vi "test Caller Stop on Last Ack.vi"(8 "error in (no error)":errorcluster, 11 "TestCase in":refnum<class "Test TCP Caller Endpoint Disconnect.lvclass">) -> (0 "error out":errorcluster, 3 "TestCase out":refnum<class "Test TCP Caller Endpoint Disconnect.lvclass">)   [LabVIEW 2020, in "Test TCP Caller Endpoint Disconnect.lvclass"]
uses:
  Test TCP Caller Endpoint Disconnect.lvclass
  <vilib>/addons/_JKI Toolkits/VI Tester/TestCase.llb/TestCase.lvclass
  <vilib>/ActorFramework/Message Queue/Message Queue.lvclass
  <vilib>/ActorFramework/LastAck/Last Ack.lvclass
  <vilib>/ActorFramework/Message Dequeuer/Message Dequeuer.lvclass
  Support/Caller Test Harness/Caller Test Harness Messages/Write String Data Msg/Write String Data Msg.lvclass
  Source/Caller Endpoint/Caller Endpoint/Caller Endpoint.lvclass
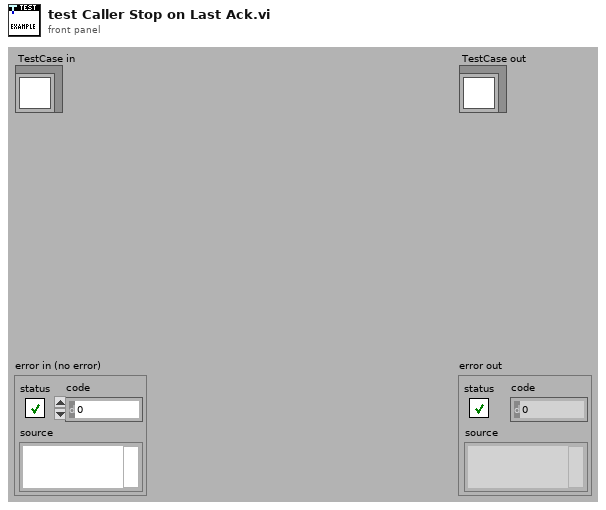
[diagram p1: front panel]
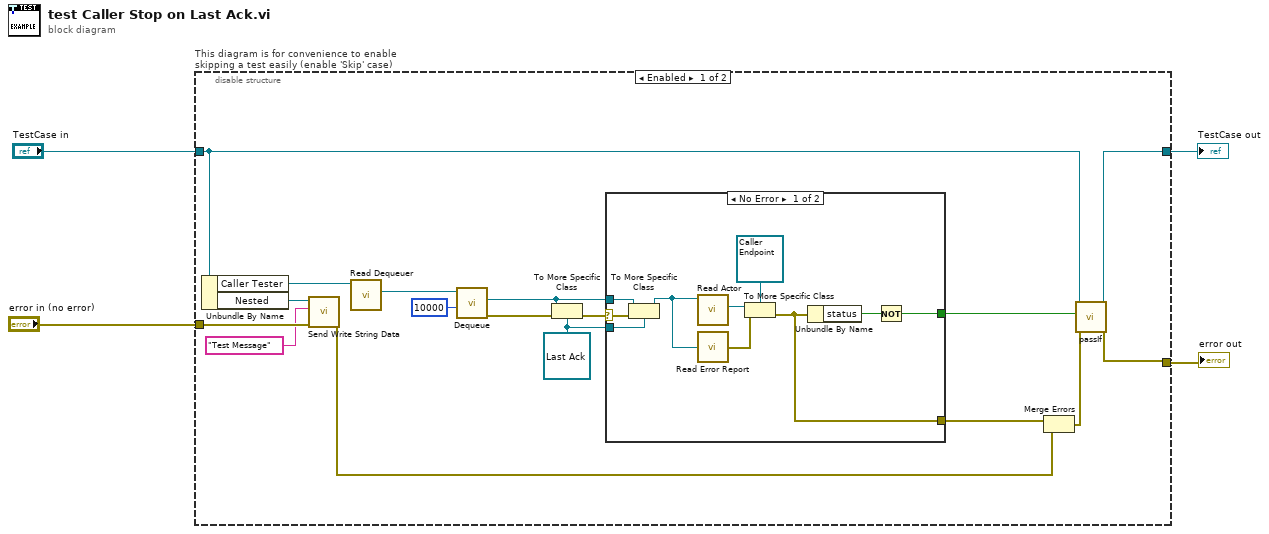
[diagram p0: block diagram]
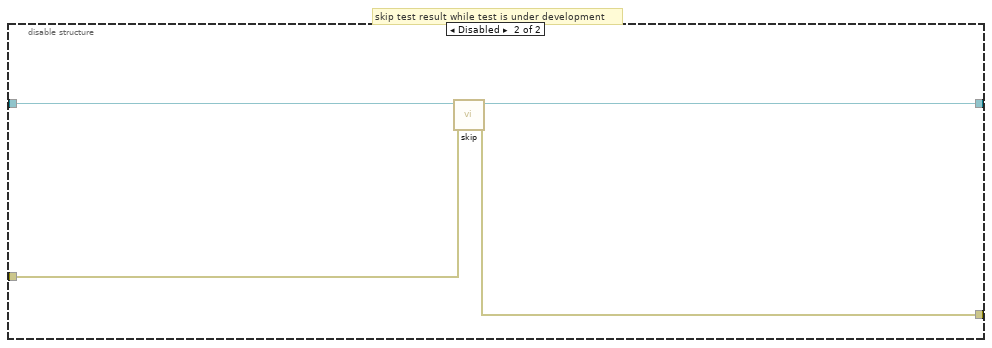
[diagram p3: hidden frame]
diagram:
  n1 = disable-structure "This diagram is for convenience to enable skipping a test easily (enable 'Skip' case)" shown="Enabled" {
    disable-tunnel: "TestCase in" -> [w19 w35]
    disable-tunnel: [w21 w33] -> w1
    disable-tunnel: [w20 w34] -> w3
    disable-tunnel: "error in (no error)" -> [w13 w32]
    frame Enabled {
      w7 = refnum<class "Last Ack.lvclass"> refnum ("Last Ack")
      n2 = Unbundle By Name(w19) -> ("Caller Tester"=w18:refnum<class "Message Queue.lvclass">, "Nested"=w14:refnum<class "Message Enqueuer.lvclass">)
      n3 = call "Send Write String Data.vi"("error in (no error)"=w13, "String Data"="Test Message", "Message Enqueuer"=w14) -> ("error out"=w12:errorcluster)  [unwired: 7 in, 1 out]
      n4 = call <vilib>:"Read Dequeuer.vi"("Message Queue"=w18) -> ("Message Dequeuer"=w16:refnum<class "Message Dequeuer.lvclass">)  [unwired: 10 in]
      n5 = call <vilib>:"Dequeue.vi"("timeout in ms (-1)"=10000, "Message Dequeuer in"=w16) -> ("error out"=w10:errorcluster, "Message"=w8:refnum<class "Message.lvclass">)  [unwired: 5 in, 3 out]
      n6 = To More Specific Class(target class=w7, reference=w8, error in=w10) -> (error out=w9:errorcluster)  [unwired: 1 out]
      n7 = case shown="No Error" w9 {
        selector: w9 -> [w30 _]
        tunnel: [w22 _] -> w6
        tunnel: [w25 _] -> w15
        tunnel: w8 -> [w29 _]
        tunnel: w7 -> [w28 _]
        frame No Error {
          n8 = To More Specific Class(target class=w28, reference=w29, error in=w30) -> (specific class reference=w27:refnum<class "Last Ack.lvclass">)  [unwired: 1 out]
          n9 = call <vilib>:"Read Actor.vi"("Last Ack"=w27) -> ("Actor"=w26:refnum<class "Actor.lvclass">)  [unwired: 10 in]
          n10 = call <vilib>:"Read Error Report.vi"("Last Ack"=w27) -> ("error report"=w24:errorcluster)
          n11 = To More Specific Class(target class=refnum<class "Caller Endpoint.lvclass"> refnum ("Caller Endpoint.lvlib:Caller Endpoint.lvclass"), reference=w26, error in=w24) -> (error out=w25:errorcluster)  [unwired: 1 out]
          n12 = Unbundle By Name(w25) -> ("status"=w31:bool)
          n13 = Not(x=w31) -> (.not. x?=w22:bool)
        }
        frame Error {
        }
      }
      n14 = Merge Errors(w15, w12) -> (w17:errorcluster)
      n15 = call-dynamic "passIf.vi"("error in (no error)"=w17, "pass"=w6, "TestCase in"=w19) -> ("error out"=w20:errorcluster, "TestCase out"=w21:refnum<class "Test TCP Caller Endpoint Disconnect.lvclass">)  [unwired: 7 in]
    }
    frame Disabled {
      # "skip test result while test is under development"
      n16 = call <vilib>:"skip.vi"("error in (no error)"=w32, "TestCase in"=w35) -> ("error out"=w34:errorcluster, "TestCase out"=w33:refnum<class "Test TCP Caller Endpoint Disconnect.lvclass">)  [unwired: 8 in]
    }
  }
  "error out" <- w3
  "TestCase out" <- w1
